vi "QuickDrop Plugin.vi"(6 "Variant in":variant, 7 "Shift Pressed?":bool, 8 "error in (no error)":errorcluster, 10 "QD Combo Box Ref":refnum<vi>, 11 "QD Launch VI Ref":refnum<vi>) -> (0 "error out":errorcluster, 4 "Variant out":variant)   [LabVIEW 2020]
doc: "Run all LUnit tests in memory which call the current VI. Hold Shift to run all tests in current project.\n\nDefault Shortcut - [L]"
uses:
  0b8230da-52ab-4c04-9608-fd4c63fdf1a3.vi
  API/LUnit Test Case/LUnit Test Case.lvclass
  C:/git/astemes-lunit/source/API/LUnit Test Case/LUnit Test Case.lvclass
  C:/git/astemes-lunit/source/Core/Runnable/Runnable.lvclass
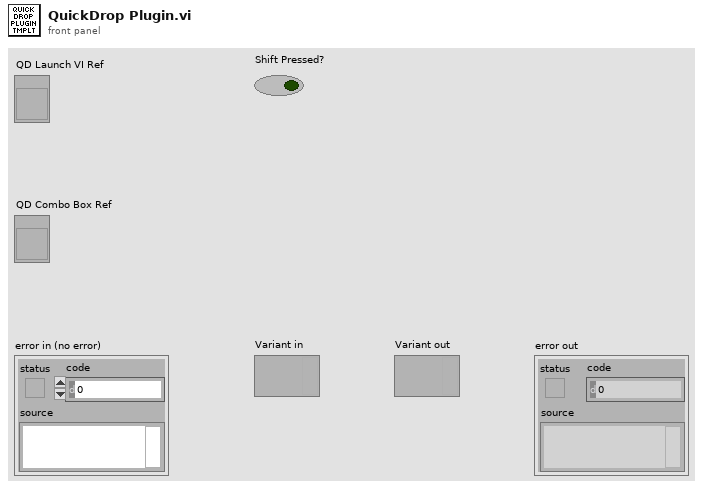
[diagram p1: front panel]
types:
  T1 = enum32{"Invalid", "Standard", "Closed", "Hidden", "Minimized", "Maximized"}
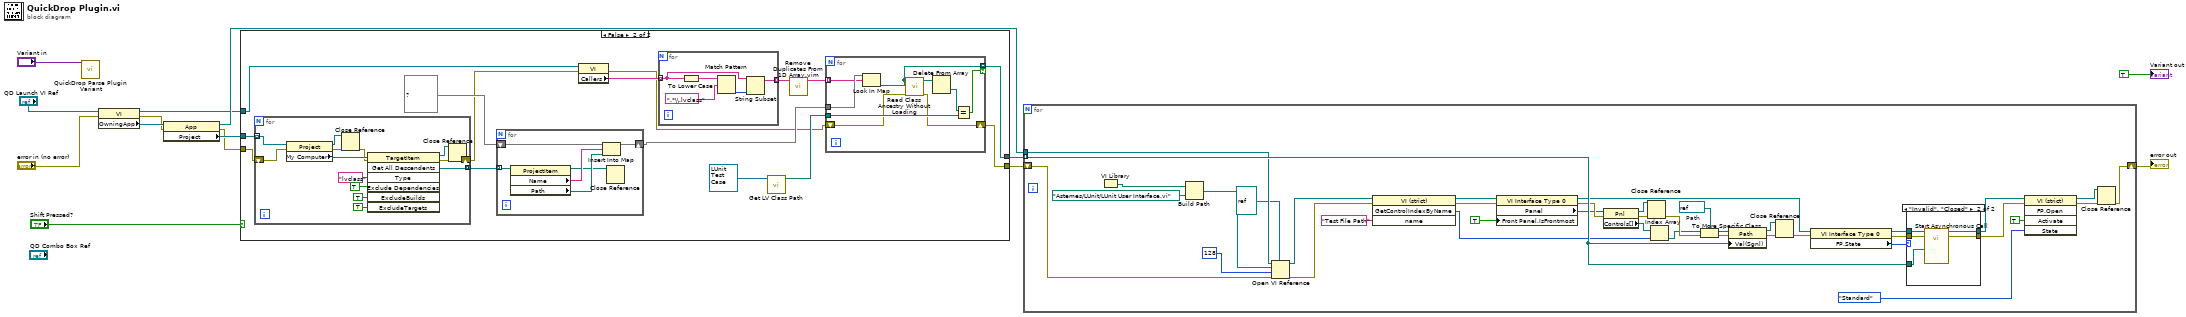
[diagram p0: block diagram]
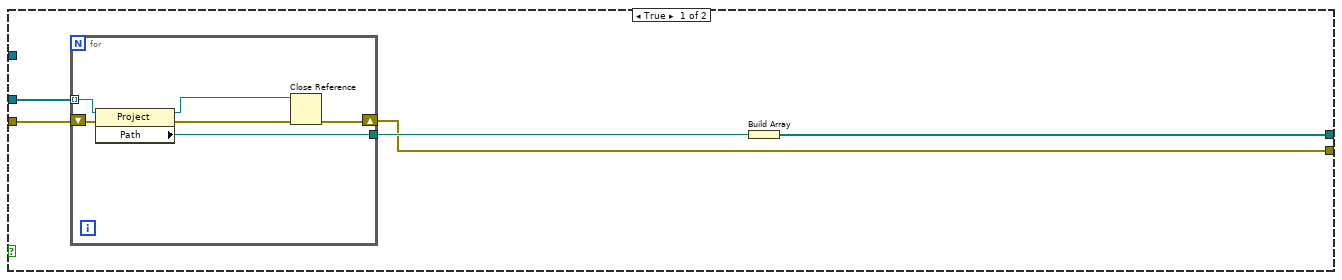
[diagram p2: hidden frame]
diagram:
  n1 = call <vilib>:"QuickDrop Parse Plugin Variant.vi"("QDKS Variant in"="Variant in") -> ()  [unwired: 12 in, 3 out]
  n2 = property class="VI"(reference="QD Launch VI Ref", error in="error in (no error)") -> (reference out=w1:refnum<vi>, error out=w6:errorcluster, "OwningApp"=w10:refnum<vi>)
  n3 = property class="App"(reference=w10, error in=w6) -> (reference out=w2:refnum<vi>, error out=w7:errorcluster, "Project"=w8:refnum<vi>[])
  n4 = case shown="False" "Shift Pressed?" {
    tunnel: w8 -> [w18 w32]
    tunnel: w7 -> [w17 w34]
    tunnel: [w16 w33] -> w5
    tunnel: [w15 w31] -> w3
    tunnel: w1 -> [_ w30]
    frame True {
      n5 = for {
        tunnel: [w25] -> w19
        tunnel: w18 -> [w21] mode=indexing
        shift-right: [w20] -> w15
        shift-left: w17 -> [w23]
        n6 = property class="Project"(reference=w21, error in=w23) -> (reference out=w22:refnum<vi>, error out=w24:errorcluster, "Path"=w25:path)
        n7 = Close Reference(reference=w22, error in (no error)=w24) -> (error out=w20:errorcluster)
      }
      n8 = Build Array(w19) -> (w16:path[])
    }
    frame False {
      n9 = for {
        tunnel: [w49] -> w40 mode=concatenating
        tunnel: w32 -> [w44] mode=indexing
        shift-right: [w42] -> w28
        shift-left: w34 -> [w47]
        n10 = property class="Project"(reference=w44, error in=w47) -> (reference out=w41:refnum<vi>, error out=w48:errorcluster, "My Computer"=w54:refnum<vi>)
        n11 = Close Reference(reference=w41, error in (no error)=w48) -> (error out=w46:errorcluster)
        n12 = invoke class="TargetItem" method="Get All Descendents"(reference=w54, error in=w46, "Type"="lvclass", "Exclude Dependencies"=TRUE ("ExcludeDependencies"), "ExcludeBuilds"=TRUE, "ExcludeTargets"=TRUE) -> (reference out=w45:refnum<vi>, error out=w43:errorcluster, "All Descendents"=w49:refnum<vi>[])  [unwired: 1 in, 4 out]
        n13 = Close Reference(reference=w45, error in (no error)=w43) -> (error out=w42:errorcluster)
      }
      n14 = for {
        tunnel: w40 -> [w60] mode=indexing
        shift-right: [w56] -> w35
        shift-left: map{string, path} {} ("map") -> [w57]
        n15 = property class="ProjectItem"(reference=w60) -> (reference out=w55:refnum<vi>, "Name"=w59:string, "Path"=w58:path)  [unwired: 1 in, 1 out]
        n16 = Insert Into Map(map in=w57, key=w59, value=w58) -> (map out=w56:map{string, path})  [unwired: 2 out]
        n17 = Close Reference(reference=w55) -> ()  [unwired: 1 in, 1 out]
      }
      n18 = property class="VI"(reference=w30, error in=w28) -> (error out=w27:errorcluster, "Callers"=w29:string[])  [unwired: 1 out]
      n19 = for {
        tunnel: w29 -> [w72] mode=indexing
        tunnel: [w71] -> w38 mode=indexing
        n20 = To Lower Case(string=w72) -> (all lower case string=w74:string)
        n21 = Match Pattern(string=w74, regular expression=".*\\.lvclass") -> (offset past match=w73:i32)  [unwired: 1 in, 3 out]
        n22 = String Subset(string=w72, length (rest)=w73) -> (substring=w71:string)  [unwired: 1 in]
      }
      n23 = call <vilib>:"Get LV Class Path.vi"("object"=refnum<class "LUnit Test Case.lvclass"> refnum ("LUnit Test Case.lvclass")) -> ("class path"=w36:path)  [unwired: 9 in, 1 out]
      n24 = call "Remove Duplicates From 1D Array.vim"("array"=w38) -> ("array with duplicates removed"=w37:string[])  [unwired: 10 in]
      n25 = for {
        tunnel: w37 -> [w64] mode=indexing
        tunnel: w36 -> [w67]
        tunnel: [w63] -> w33 mode=indexing if=w66
        tunnel: w35 -> [w65]
        shift-right: [w62] -> w31
        shift-left: w27 -> [w61]
        n26 = Look In Map(map=w65, key=w64) -> (value=w63:path)  [unwired: 1 in, 1 out]
        n27 = call <vilib>:"Read Class Ancestry Without Loading.vi"("error in (no error)"=w61, "LabVIEW Class Path"=w63) -> ("error out"=w62:errorcluster, "Class Ancestry"=w69:path[])  [unwired: 8 in]
        n28 = Delete From Array(array=w69) -> (deleted portion=w68:path)  [unwired: 2 in, 1 out]
        n29 = Equal?(x=w68, y=w67) -> (x = y?=w66:bool)
      }
    }
  }
  n30 = for {
    tunnel: w5 -> [w113] mode=indexing
    tunnel: w2 -> [w112]
    shift-right: [w111] -> w4
    shift-left: w3 -> [w110]
    w89 = refnum<vi> refnum  # Path
    n31 = VI Library() -> (path=w83:path)
    n32 = Build Path(base path=w83, name or relative path=path "Astemes/LUnit/LUnit User Interface.vi" ("Relative Path from 1 to 2")) -> (appended path=w78:path)
    n33 = Open VI Reference(type specifier VI Refnum (for type only)=refnum<vi> refnum, application reference (local)=w112, vi path=w78, options=128, error in (no error)=w110) -> (vi reference=w101:refnum<vi>, error out=w102:errorcluster)  [unwired: 1 in]
    n34 = invoke class="VI (strict)" method="GetControlIndexByName"(reference=w101, error in=w102, "name"="Test File Path" ("Control Name")) -> (reference out=w85:refnum<vi>, error out=w95:errorcluster, "GetControlIndexByName"=w88:i32)  [unwired: 1 in, 1 out]
    n35 = property class="VI Interface Type 0"(reference=w85, error in=w95, "Front Panel.IsFrontmost"=TRUE ("Front Panel Window:Is Frontmost")) -> (reference out=w108:refnum<vi>, error out=w94:errorcluster, "Panel"=w84:refnum<vi>)
    n36 = property class="Pnl"(reference=w84, error in=w94) -> (reference out=w98:refnum<vi>, error out=w93:errorcluster, "Controls[]"=w87:refnum<vi>[])
    n37 = Close Reference(reference=w98, error in (no error)=w93) -> (error out=w97:errorcluster)
    n38 = Index Array(array=w87, index=w88) -> (element=w91:refnum<vi>)
    n39 = To More Specific Class(target class=w89, reference=w91, error in=w97) -> (specific class reference=w90:refnum<vi>, error out=w92:errorcluster)
    n40 = property class="Path"(reference=w90, error in=w92, "Val(Sgnl)"=w113) -> (reference out=w99:refnum<vi>, error out=w96:errorcluster)
    n41 = Close Reference(reference=w99, error in (no error)=w96) -> (error out=w106:errorcluster)
    n42 = property class="VI Interface Type 0"(reference=w108, error in=w106) -> (reference out=w104:refnum<vi>, error out=w103:errorcluster, "FP.State"=w105:T1)
    n43 = case shown="\"Invalid\", \"Closed\"" w105 {
      tunnel: w103 -> [w115 w120]
      tunnel: w104 -> [w114 w119]
      tunnel: [w115 w117] -> w107
      tunnel: [w114 w118] -> w109
      tunnel: w113 -> [_ w116]
      frame Default {
      }
      frame "Invalid", "Closed" {
        n44 = call-by-ref "Start Asynchronous Call"(reference=w119, error in=w120, "Test File Path"=w116) -> (reference out=w118:refnum<vi>, error out=w117:errorcluster)  [unwired: 11 in]
      }
    }
    n45 = invoke class="VI (strict)" method="FP.Open"(reference=w109, error in=w107, "Activate"=TRUE ("Activate?"), "State"=T1."Standard") -> (reference out=w79:refnum<vi>, error out=w80:errorcluster)  [unwired: 1 in, 3 out]
    n46 = Close Reference(reference=w79, error in (no error)=w80) -> (error out=w111:errorcluster)
  }
  "error out" <- w4
  "Variant out" <- TRUE
